vi "Frequenzmessung vervielfachen.vi"(9 "true=mehrfach Messen":bool, 10 "Anzahl der Messungen bei einer Frequenz":i32=10, 11 "Eingang":T1(array[cluster])) -> (3 "Ausgang":T1(graph))   [LabVIEW 2018]
panel:
  out "Ausgangsliste":T1(array[cluster])
  out "Eingangsliste":T1(graph)
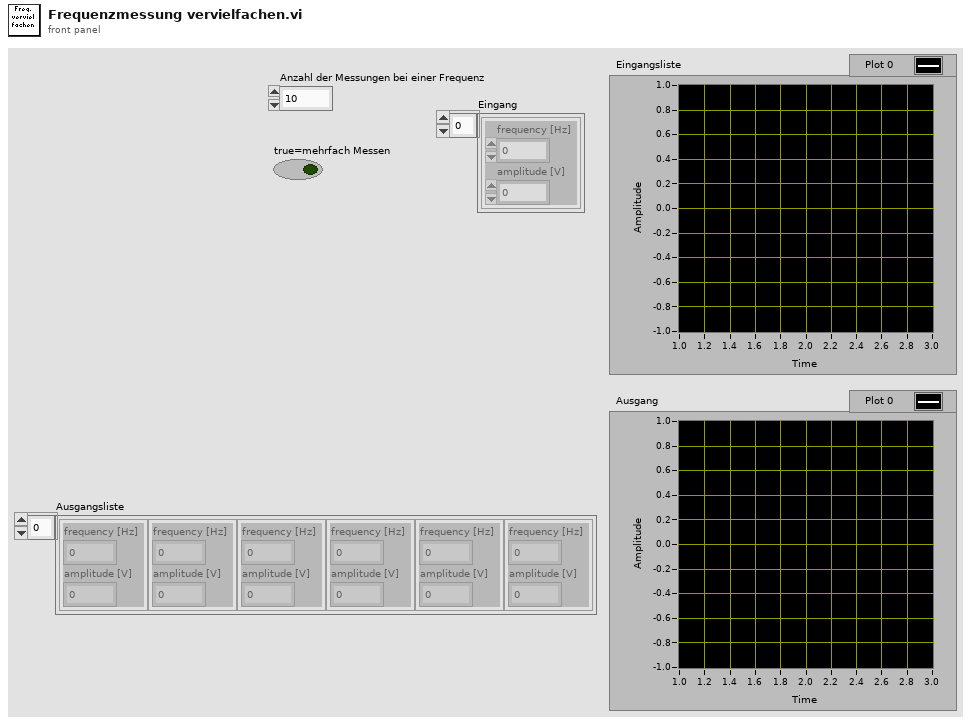
[diagram p1: front panel]
types:
  T1 = cluster{"frequency [Hz]":dbl, "amplitude [V]":dbl}[]
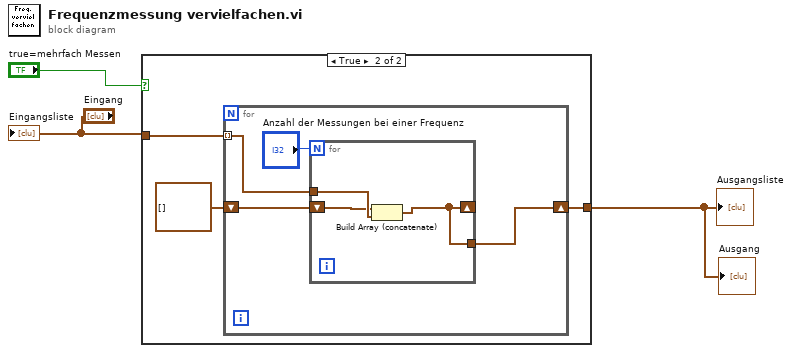
[diagram p0: block diagram]
diagram:
  n1 = case shown="True" "true=mehrfach Messen" {
    tunnel: "Eingang" -> [w4 w7]
    tunnel: [w4 w6] -> w2
    frame False {
    }
    frame True {
      n2 = for {
        tunnel: w7 -> [w10] mode=indexing
        shift-right: [w9] -> w6
        shift-left: T1 [] -> [w8]
        n3 = for {
          N: "Anzahl der Messungen bei einer Frequenz" -> [_]
          tunnel: w10 -> [w14]
          shift-right: [w12] -> _
          shift-left: w8 -> [w13]
          tunnel: [w12] -> w9
          n4 = Build Array (concatenate)(w13, w14) -> (w12:T1)
        }
      }
    }
  }
  "Ausgangsliste" <- w2
  "Ausgang" <- w2
  "Eingangsliste" <- "Eingang"
